vi "Return Acquisition Mode.vi"(10 "Acquisition Mode":string) -> (3 "Multiply Factor":i32)   [LabVIEW 2020, in "Agilent 90000 Series.lvlib"]
doc: "Returns the mutiply factor based on the acquistion mode."
uses:
  Agilent 90000 Series.lvlib
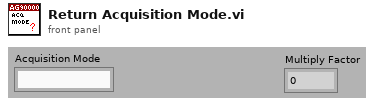
[diagram p1: front panel]
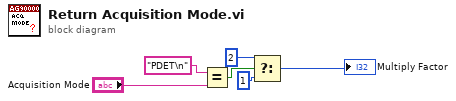
[diagram p0: block diagram]
diagram:
  n1 = Equal?(x="PDET\n", y="Acquisition Mode") -> (x = y?=w6:bool)
  n2 = Select(t=2, s=w6, f=1) -> (s? t:f=→"Multiply Factor":i32)
